vi "Central Error Handler Template(RT).vi"   [LabVIEW 2014]
doc: "This VI provides a template from which to build a Central Error Handler that is capable of receiving and responding to error notifications from specific error handlers. The Central Error Handler is responsible for taking actions which cannot or should not be performed in-line with executing code such as:\n- Error logging\n- Initiating a safe state\n- Shutting down the system\n- Notifying an HMI\n\nThis VI is optimized for Real-Time applications. An alternate version for Windows VIs exists."
uses:
  Controls/CEH/CEH Actions.ctl
types:
  T1 = typedef "SEH Notification Info.ctl" = cluster{"Priority":i32, "Occurrences":i32, "First Occurrence":timestamp}
  T2 = typedef "CEH Actions.ctl" = enum16{"Log", "Display Error Message", "Safe State", "Shutdown"}
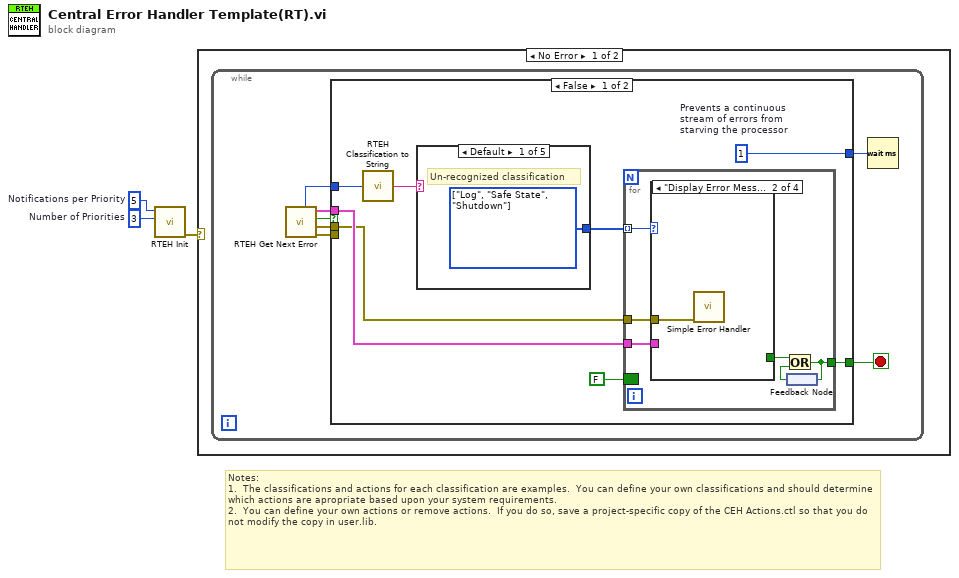
[diagram p0: block diagram]
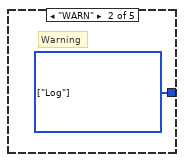
[diagram p2: hidden frame]
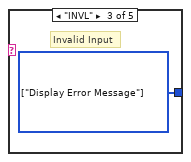
[diagram p3: hidden frame]
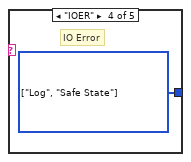
[diagram p4: hidden frame]
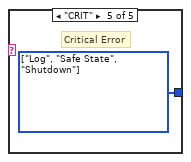
[diagram p5: hidden frame]
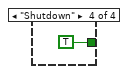
[diagram p8: hidden frame]
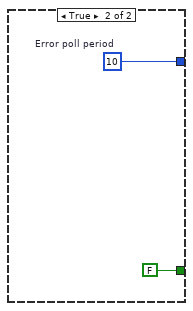
[diagram p9: hidden frame]
diagram:
  w2 = 3  # Number of Priorities
  w3 = 5  # Notifications per Priority
  # "Notes:\n1.  The classifications and actions for each classification are examples.  You can define your own classifications and should determine which actions are apropriate based upon your system requirements.\n2.  You can define your own actions or remove actions.  If you do so, save a project-specific copy of the CEH Actions.ctl so that you do not modify the copy in user.lib."
  n1 = call "RTEH Init.vi"("Number of Priorities"=w2, "Notifications per Priority"=w3) -> ("error out"=w1:errorcluster)  [unwired: 9 in]
  n2 = case shown="No Error" w1 {
    frame No Error {
      n3 = while {
        stop <- w9 stop-if-true
        n4 = call "RTEH Get Next Error.vi"() -> ("Internal Error"=w5:errorcluster, "Transmitted Error"=w8:errorcluster, "Empty?"=w7:bool, "Notification Info"=w6:T1, "Classification"=w4:u32)  [unwired: 7 in]
        n5 = case shown="False" w7 {
          tunnel: [w18 w33] -> w10
          tunnel: w8 -> [w13 _]
          tunnel: w6 -> [w16 _]
          tunnel: [w15 FALSE] -> w9
          tunnel: w5 -> [_ _]
          tunnel: w4 -> [w11 _]
          frame False {
            w18 = u32 1  # Prevents a continuous stream of errors from starving the processor
            n6 = call "RTEH Classification to String.vi"("Classification as Number"=w11) -> ("Classification as String"=w12:string)  [unwired: 14 in]
            n7 = case shown="Default" w12 {
              tunnel: [w19 w20 w21 w22 w23] -> w17
              frame Default {
                w19 = T2[] [enum."Log", enum."Safe State", enum."Shutdown"] items=["Log", "Display Error Message", "Safe State", "Shutdown"]
                # "Un-recognized classification"
              }
              frame "WARN" {
                w20 = T2[] [enum."Log"] items=["Log", "Display Error Message", "Safe State", "Shutdown"]
                # "Warning"
              }
              frame "INVL" {
                w21 = T2[] [enum."Display Error Message"] items=["Log", "Display Error Message", "Safe State", "Shutdown"]
                # "Invalid Input"
              }
              frame "IOER" {
                w22 = T2[] [enum."Log", enum."Safe State"] items=["Log", "Display Error Message", "Safe State", "Shutdown"]
                # "IO Error"
              }
              frame "CRIT" {
                w23 = T2[] [enum."Log", enum."Safe State", enum."Shutdown"] items=["Log", "Display Error Message", "Safe State", "Shutdown"]
                # "Critical Error"
              }
            }
            n8 = for {
              tunnel: w13 -> [w28]
              tunnel: w17 -> [w29] mode=indexing
              tunnel: w16 -> [w27]
              border: FALSE -> [_]
              tunnel: [w24] -> w15
              n9 = case shown="\"Display Error Message\"" w29 {
                tunnel: w28 -> [_ w30 _ _]
                tunnel: w27 -> [_ _ _ _]
                tunnel: [_ _ _ TRUE] -> w26
                frame "Log", Default {
                }
                frame "Display Error Message" {
                  n10 = call <vilib>:"Simple Error Handler.vi"("error in (no error)"=w30) -> ()  [unwired: 4 in, 5 out]
                }
                frame "Safe State" {
                }
                frame "Shutdown" {
                }
              }
              n11 = feedback #1() -> (w25:bool)
              n12 = Or(x=w26, y=w25) -> (x .or. y?=w24:bool)
              n13 = feedback-in #1(w24) -> ()
            }
          }
          frame True {
            w33 = u32 10  # Error poll period
          }
        }
        n14 = Wait (ms)(milliseconds to wait=w10) -> ()  [unwired: 1 out]
      }
    }
    frame Error {
      # "Error notification cannot initialize\n(log this)"
    }
  }
